vi "test serial.vi"() -> ()   [LabVIEW 2016]
panel:
  in  "connection parameters":T1={"baud rate (9600)"=9600, "data bits (8)"=8, "stop bits (10: 1 bit)"=10, "parity (0:none)"=enum."None", "flow control (0:none)"=0, "timeout (10sec)"=10000, "Enable Termination\nChar (T)"=TRUE, "termination char\n(0xA = '\\n' = LF)\n(0xD = '\\r' = CF) "=13} {"flow control (0:none)" items=["None", "XON/XOFF", "RTS/CTS", "XON/XOFF & RTS/CTS", "DTR/DSR", "XON/XOFF & DTR/DSR"]; "stop bits (10: 1 bit)" items=["1.0"=10, "1.5"=15, "2.0"=20]}
  out "read buffer":string
  in  "stop":bool
  in  "update":bool
  in  "write buffer":string
  in  "port name in":refnum<visa-resource-name>
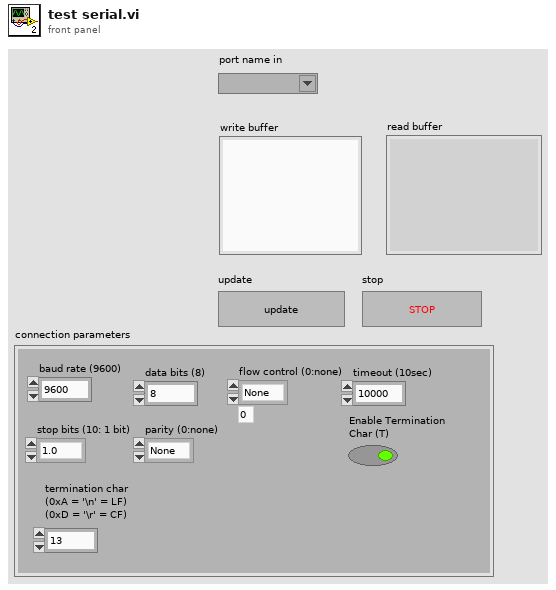
[diagram p1: front panel]
types:
  T1 = cluster{"baud rate (9600)":u32, "data bits (8)":u16, "stop bits (10: 1 bit)":u16, "parity (0:none)":enum16{"None", "Odd", "Even", "Mark", "Space"}, "flow control (0:none)":u16, "timeout (10sec)":u32, "Enable Termination\nChar (T)":bool, "termination char\n(0xA = '\\n' = LF)\n(0xD = '\\r' = CF) ":u8}
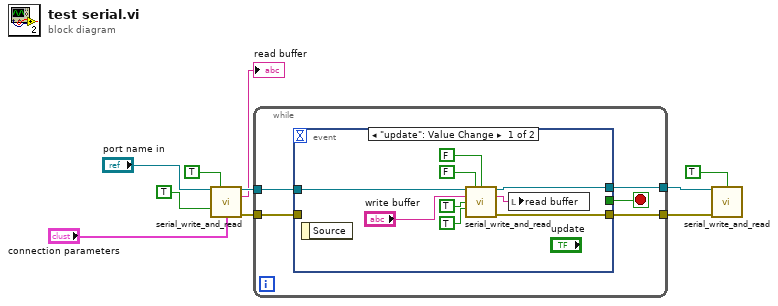
[diagram p0: block diagram]
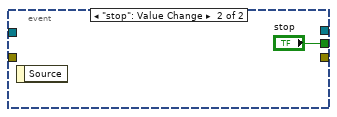
[diagram p2: hidden frame]
diagram:
  n1 = call "serial_write_and_read.vi"("port name in"="port name in", "reconnect?"=TRUE, "expecting response?"=TRUE, "connection parameters"="connection parameters") -> ("port name out"=w7:refnum<visa-resource-name>, "read buffer"=→"read buffer":string, "error out"=w8:errorcluster)  [unwired: 9 in]
  n2 = while {
    tunnel: w8 -> [w15]
    tunnel: w7 -> [w14]
    tunnel: [w13] -> w6
    tunnel: [w12] -> w4
    stop <- w11 stop-if-true
    n3 = event shown="[0] \"update\": Value Change" {
      selector: _ -> [_ _]
      dyn-events: _ -> [_ _]
      timeout: _ -> [_ _]
      tunnel: w15 -> [_ _]
      tunnel: w14 -> [w24 _]
      tunnel: [w23 _] -> w13
      tunnel: [w22 _] -> w12
      tunnel: [_ "stop"] -> w11
      event "update": Value Change {
        n4 = event-data() -> ()  [unwired: 1 in, 1 out]
        n5 = call "serial_write_and_read.vi"("port name in"=w24, "reconnect?"=FALSE, "disconnect?"=FALSE, "write buffer"="write buffer", "do writing?"=TRUE, "expecting response?"=TRUE) -> ("port name out"=w23:refnum<visa-resource-name>, "read buffer"=w18:string, "error out"=w22:errorcluster)  [unwired: 7 in]
        n6 = local write "read buffer"(w18) -> ()
      }
      event "stop": Value Change {
        n7 = event-data() -> ()  [unwired: 1 in, 1 out]
      }
    }
  }
  n8 = call "serial_write_and_read.vi"("port name in"=w6, "disconnect?"=TRUE, "error in"=w4) -> ()  [unwired: 10 in, 3 out]
